vi "Insight_Calibrate_Fixed_Wavelength_Power.vi"(8 "error in (no error)":errorcluster, 11 "telnet connection":T1) -> (0 "error out":errorcluster, 1 "response data":string, 3 "telnet  connection out":T1)   [LabVIEW 2015]
doc: "Insight Photonic Solutions\n\nThis calibrates the power of the laser in Fixed Wavelength Mode. If you change the power, you need to run Power Calibration in Fixed Wavelength Mode to assure that all wavelengths are at the new power level.\n\nInputs:\nRead/Write : command or query the state of Fixed Wavelength Mode\n\nOutputs:\nResponse Data - Entire string response from the laser\n\nver 1.0 - original release"
uses:
  Telnet Session.ctl
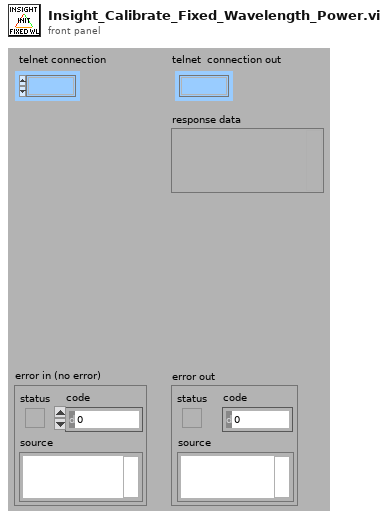
[diagram p1: front panel]
types:
  T1 = typedef "Telnet Session.ctl" = refnum<k1>
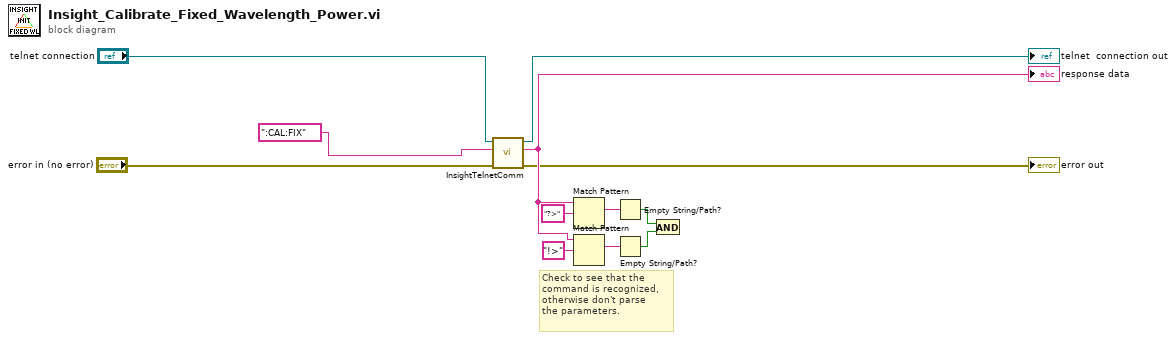
[diagram p0: block diagram]
diagram:
  # "Check to see that the \ncommand is recognized,\notherwise don't parse \nthe parameters."
  n1 = call "InsightTelnetComm.vi"("error in"="error in (no error)", "write buffer (\"\")"=":CAL:FIX" ("String"), "telnet connection"="telnet connection") -> ("error out"=→"error out":errorcluster, "response data"=w4:string, "telnet  connection out"=→"telnet  connection out":T1)  [unwired: 4 in]
  "response data" <- w4
  n2 = Match Pattern(string=w4, regular expression="?>") -> (match substring=w9:string)  [unwired: 1 in, 3 out]
  n3 = Match Pattern(string=w4, regular expression="!>") -> (match substring=w8:string)  [unwired: 1 in, 3 out]
  n4 = Empty String/Path?(string/path=w9) -> (empty?=w6:bool)
  n5 = Empty String/Path?(string/path=w8) -> (empty?=w5:bool)
  n6 = And(x=w6, y=w5) -> ()  [unwired: 1 out]
